vi "Get Size.vi"(8 "error in (no error)":errorcluster, 11 "Picture Control Canvas in":refnum<class "Picture Control Canvas.lvclass">) -> (0 "error out":errorcluster, 2 "Size":cluster{"Width":u16, "Height":u16}, 3 "Picture Control Canvas out":refnum<class "Picture Control Canvas.lvclass">)   [LabVIEW 2020, in "Glyph Drawer.lvlib" / "Picture Control Canvas.lvclass"]
uses:
  Picture Control Canvas.lvclass
  Picture Control Canvas.lvclass/Picture Control Canvas.ctl
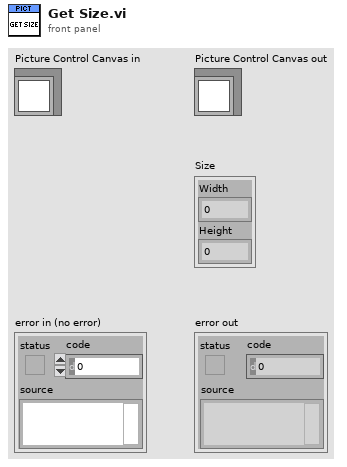
[diagram p1: front panel]
types:
  T1 = typedef "LVBoundsTypeDef.ctl" = cluster{"Width":u32, "Height":u32}
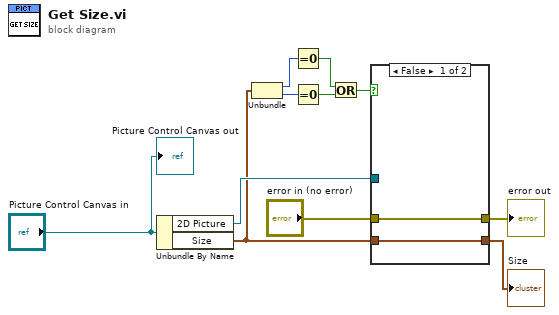
[diagram p0: block diagram]
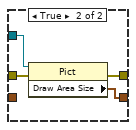
[diagram p2: hidden frame]
diagram:
  n1 = Unbundle By Name("Picture Control Canvas in") -> ("2D Picture"=w10:refnum<vi>, "Size"=w1:cluster{"Width":u16, "Height":u16})
  n2 = Unbundle(w1) -> ("Width"=w6:u16, "Height"=w4:u16)
  n3 = Equal To 0?(x=w6) -> (x = 0?=w2:bool)
  n4 = Equal To 0?(x=w4) -> (x = 0?=w5:bool)
  n5 = Or(x=w2, y=w5) -> (x .or. y?=w3:bool)
  n6 = case shown="False" w3 {
    tunnel: w10 -> [_ w17]
    tunnel: [w13 w16] -> w9
    tunnel: "error in (no error)" -> [w12 w15]
    tunnel: [w12 w14] -> w7
    tunnel: w1 -> [w13 _]
    frame False {
    }
    frame True {
      n7 = property class="Pict"(reference=w17, error in=w15) -> (error out=w14:errorcluster, "Draw Area Size"=w16:T1)  [unwired: 1 out]
    }
  }
  "error out" <- w7
  "Size" <- w9
  "Picture Control Canvas out" <- "Picture Control Canvas in"
